vi "Close.vi"(8 "Error In (No Error)":errorcluster, 11 "RS232 Port In":refnum<visa-resource-name>) -> (0 "Error Out":errorcluster)   [LabVIEW 2016, in "SDI-12.lvlib"]
doc: "Closes the VISA Reference to the serial port that is connected to the RS232 to SDI-12 converter. This VI should be called before an application finishes."
uses:
  SDI-12.lvlib
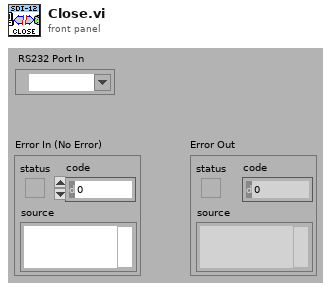
[diagram p1: front panel]
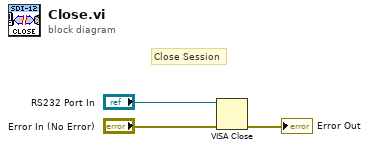
[diagram p0: block diagram]
diagram:
  # "Close Session"
  n1 = VISA Close(VISA resource name="RS232 Port In", error in (no error)="Error In (No Error)") -> (error out=→"Error Out":errorcluster)
